vi "Last Ack Creator.vi"(10 "jettl":refnum<class "jettl.lvclass">, 11 "Base jettl in":refnum<class "Base jettl.lvclass">) -> (3 "Base jettl out":refnum<class "Base jettl.lvclass">)   [LabVIEW 2021, in "jettl.lvlib" / "Base jettl.lvclass"]
uses:
  Base jettl.lvclass
  jettl/jettl.lvclass
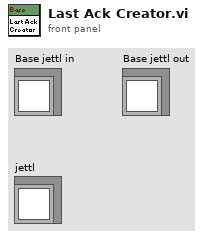
[diagram p1: front panel]
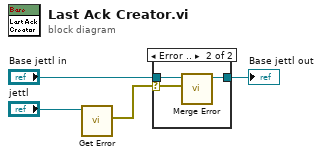
[diagram p0: block diagram]
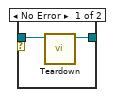
[diagram p2: hidden frame]
diagram:
  n1 = call-dynamic "Get Error.vi"("jettl in"="jettl") -> ("Error"=w4:errorcluster)  [unwired: 10 in]
  n2 = case shown="Error .." w4 {
    selector: w4 -> [_ w9]
    tunnel: "Base jettl in" -> [w6 w8]
    tunnel: [w5 w7] -> w2
    frame No Error {
      n3 = call-dynamic "Teardown.vi"("Base jettl in"=w6) -> ("Base jettl out"=w5:refnum<class "Base jettl.lvclass">)  [unwired: 10 in]
    }
    frame Error {
      n4 = call-dynamic "Merge Error.vi"("Error"=w9, "Base jettl in"=w8) -> ("Base jettl out"=w7:refnum<class "Base jettl.lvclass">)  [unwired: 9 in]
    }
  }
  "Base jettl out" <- w2
